vi "onDisconnection.vi"(8 "error in (no error)":errorcluster, 11 "LocalQueueConnection in":refnum<class "LocalQueueConnection.lvclass">) -> (0 "error out":errorcluster, 3 "No Connection":refnum<class "LocalQueueConnection.lvclass">)   [LabVIEW 2013, in "MQTT_Queue.lvlib" / "LocalQueueConnection.lvclass"]
uses:
  LocalQueueConnection.lvclass
  <vilib>/LabVIEW Open Source Project/MQTT Connection/MQTT_Connection/Connection/Connection.lvclass
  LocalQueueConnection.lvclass/LocalQueueConnection.ctl
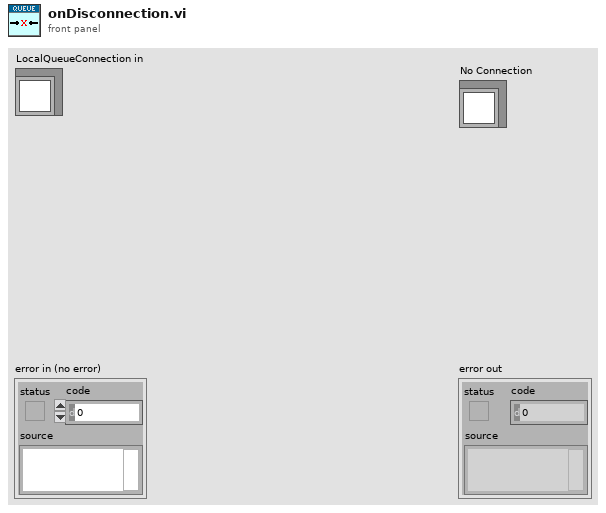
[diagram p1: front panel]
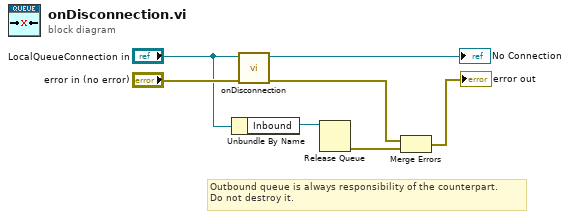
[diagram p0: block diagram]
diagram:
  # "Outbound queue is always responsibility of the counterpart.\nDo not destroy it."
  n1 = Unbundle By Name("LocalQueueConnection in") -> ("Inbound"=w2:refnum<queue>)
  n2 = call-parent "onDisconnection.vi"("error in (no error)"="error in (no error)", "Connection"="LocalQueueConnection in") -> ("error out"=w5:errorcluster, "No connection"=→"No Connection":refnum<class "LocalQueueConnection.lvclass">)  [unwired: 8 in]
  n3 = Release Queue(queue=w2) -> (error out=w1:errorcluster)  [unwired: 2 in, 2 out]
  n4 = Merge Errors(w5, w1) -> (→"error out":errorcluster)
